vi "Init.vi"(0 "I2C Bus":T1=enum."Invalid", 5 "Device Address":u8 format="%.0x", 11 "error in":errorcluster) -> (4 "comm interface out":refnum<class "Pixy Com.lvclass">, 15 "error out":errorcluster)   [LabVIEW 2018, in "RoboRIO I2C.lvclass"]
doc: "Initializes a Pixy2 communication session for the RoboRIO I2C bus."
uses:
  RoboRIO I2C.lvclass
  <vilib>/Rock Robotics/SystemInterfaces/i2clib/i2c_bus.ctl
  library/Interface/Pixy Com.lvclass
  C:/Users/David/Documents/GitHub/Pixy2LabVIEW/source/Interface/Pixy Com.lvclass
  RoboRIO I2C.lvclass/RoboRIO I2C.ctl
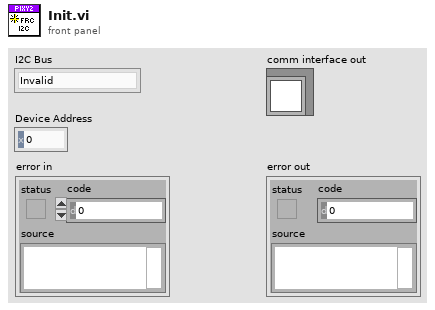
[diagram p1: front panel]
types:
  T1 = typedef "i2c_bus.ctl" = enum16{"I2C On-Board", "I2C MXP", "Invalid"}
  T2 = typedef "WPI_I2CDevRef.ctl" = cluster{"DevStatus":errorcluster, "Device Address":u8, "Handle":i32, "I2C Bus":T1}
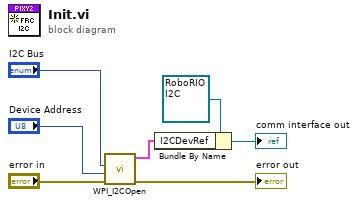
[diagram p0: block diagram]
diagram:
  n1 = call <vilib>:"WPI_I2COpen.vi"("error in"="error in", "Device Address"="Device Address", "I2C Bus"="I2C Bus") -> ("error out"=→"error out":errorcluster, "I2CDevRef"=w2:T2)  [unwired: 7 in]
  n2 = Bundle By Name(cluster=refnum<class "RoboRIO I2C.lvclass"> refnum, "I2CDevRef"=w2) -> (→"comm interface out":refnum<class "RoboRIO I2C.lvclass">)
